vi "Main Engine Get Hardware Info.vi"(8 "error in":errorcluster) -> (0 "error out":errorcluster, 1 "CPU Session":refnum<k21>, 2 "IPAddress":string, 3 "Hardware Info":T3[](array[typedef]) {"Is Present?" items=["Initializing"=-2, "Unknown"=-1, "Not Present"=0, "Present"=1]}, 4 "DAQ Device Info":T1[](array[typedef]), 5 "Serial Device Info":T2[](array[typedef]), 6 "Ethernet IP Address":string[](array[string]), 7 "CPU Ref":refnum<k20>)   [LabVIEW 2021]
doc: "Get cRIO Info\n\n\nAll Rights Reserved © 2023 SyncSols"
uses:
  Controls/Main Engine Hardware Info Data Cluster.ctl
  Controls/Main Engine Serial Card Details.ctl
  Controls/Main Engine DAQ Device Info.ctl
  <vilib>/Instr/_visa.llb/VISA Find Search Mode.ctl
  <userlib>/_OpenG.lib/array/array.llb/Remove Duplicates from 1D Array (String)__ogtk.vi
  <vilib>/nisyscfg/nisyscfg.lvlib
  <resource>/objmgr/nicriosae.rc
  <resource>/objmgr/daqmx.rc
  <userlib>/_OpenG.lib/array/array.llb/openg_array.lvlib
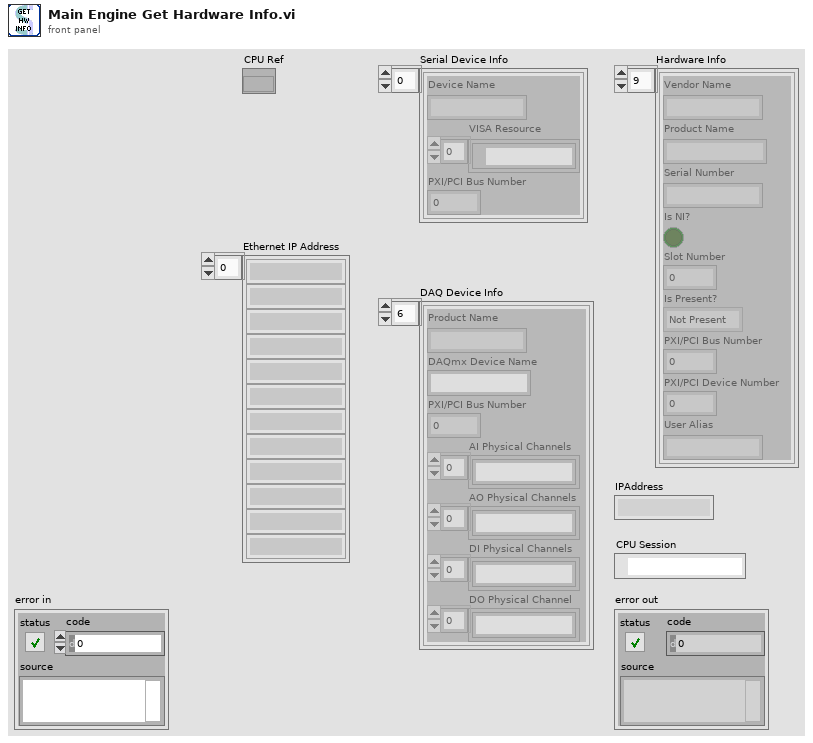
[diagram p1: front panel]
types:
  T1 = typedef "Main Engine DAQ Device Info.ctl" = cluster{"Product Name":string, "DAQmx Device Name":string, "PXI/PCI Bus Number":u32, "AI Physical Channels":string[], "AO Physical Channels":string[], "DI Physical Channels":string[], "DO Physical Channel":string[]}
  T2 = typedef "Main Engine Serial Card Details.ctl" = cluster{"Device Name":string, "VISA Resource":refnum<visa-resource-name>[], "PXI/PCI Bus Number":u32}
  T3 = typedef "Main Engine Hardware Info Data Cluster.ctl" = cluster{"Vendor Name":string, "Product Name":string, "Serial Number":string, "Is NI?":bool, "Slot Number":i32, "Is Present?":i32, "PXI/PCI Bus Number":u32, "PXI/PCI Device Number":u32, "User Alias":string}
  T4 = typedef "VISA Find Search Mode.ctl" = u32
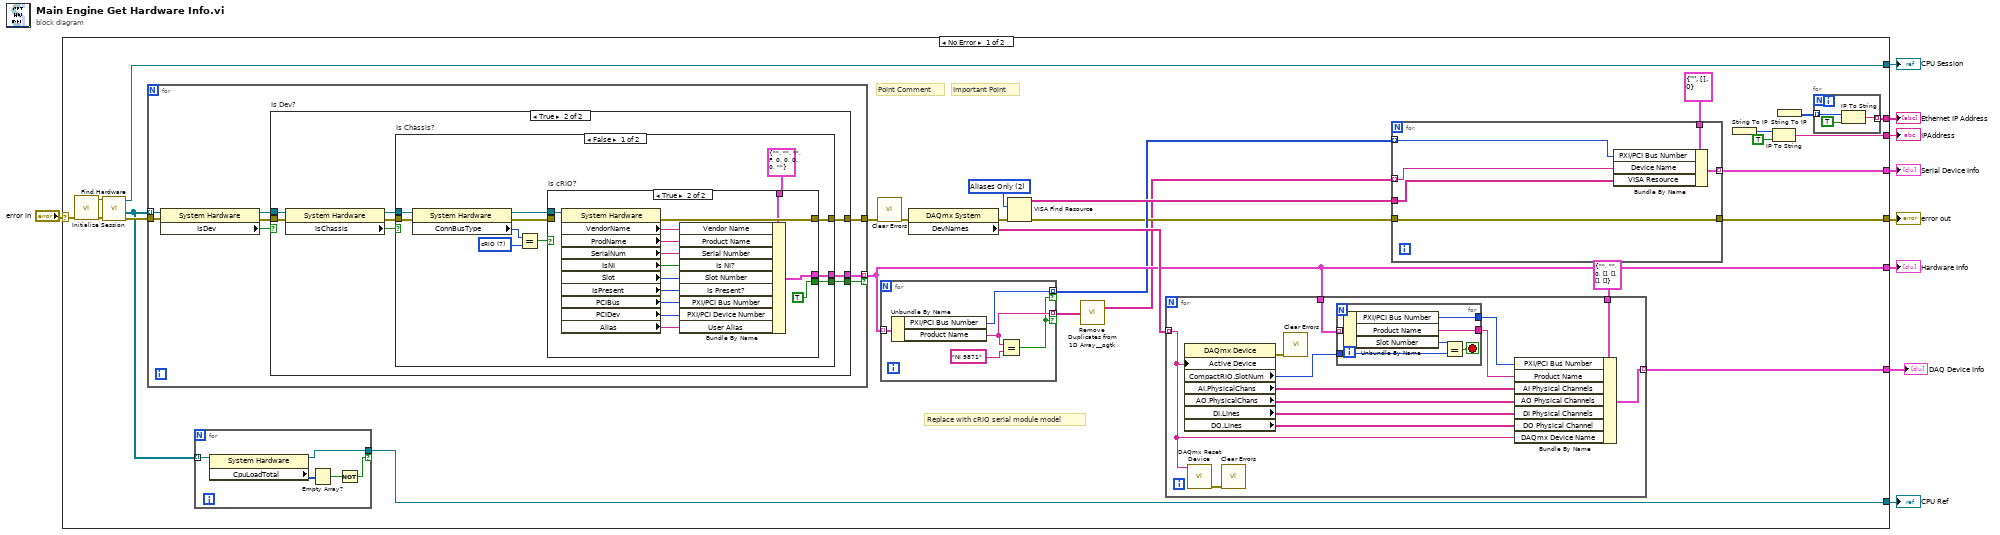
[diagram p0: block diagram]
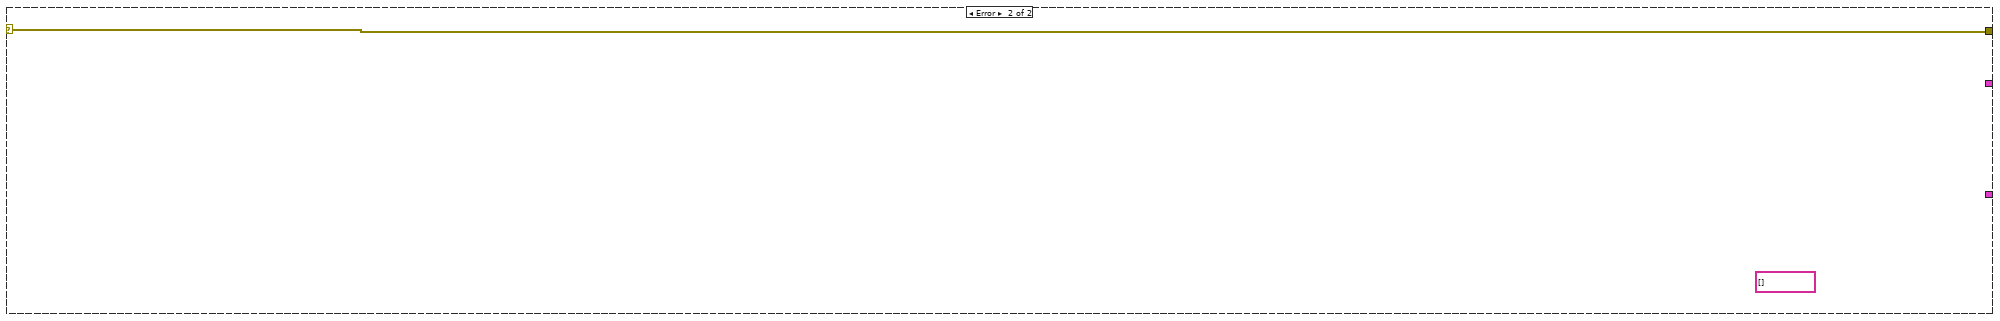
[diagram p5: hidden frame]
diagram:
  n1 = case shown="No Error" "error in" {
    selector: "error in" -> [w35 w120]
    tunnel: [w26 w120] -> w9
    tunnel: [w24 _] -> w7
    tunnel: [w33 _] -> w6
    tunnel: [w27 _] -> w5
    tunnel: [w23 _] -> w4
    tunnel: [w16 _] -> w3
    tunnel: [w15 _] -> w1
    tunnel: [w13 _] -> w2
    frame No Error {
      w29 = T4 2 items=["Canonical Names Only"=0, "Aliases Only"=2, "Include Matching Aliases"=3, "Include All Aliases"=4] ("Search Mode")
      # "Replace with cRIO serial module model"
      # "Important Point"
      # "Point Comment"
      n2 = call <vilib>:"Initialize Session.vi"("error in (no error)"=w35) -> ("error out"=w37:errorcluster, "Session out"=w36:refnum<k21>)  [unwired: 9 in]
      n3 = call <vilib>:"Find Hardware.vi"("error in (no error)"=w37, "Session in"=w36) -> ("error out"=w34:errorcluster, "Resources out"=w14:refnum<k20>[], "Session out"=w15:refnum<k21>)  [unwired: 6 in, 1 out]
      n4 = for {
        tunnel: w14 -> [w83] mode=indexing
        tunnel: w34 -> [w79]
        tunnel: [w78] -> w31
        tunnel: [w77] -> w24 mode=indexing if=w76
        n5 = property class="System Hardware"(reference=w83, error in=w79) -> (reference out=w82:refnum<k20>, error out=w81:errorcluster, "IsDev"=w80:bool)
        n6 = case "Is Dev?" shown="True" w80 {
          tunnel: w82 -> [_ w92]
          tunnel: w81 -> [w84 w91]
          tunnel: [w84 w87] -> w78
          tunnel: [_ w86] -> w76
          tunnel: [_ w85] -> w77
          frame False {
          }
          frame True {
            n7 = property class="System Hardware"(reference=w92, error in=w91) -> (reference out=w90:refnum<k20>, error out=w88:errorcluster, "IsChassis"=w89:bool)
            n8 = case "Is Chassis?" shown="False" w89 {
              tunnel: w90 -> [w103 _]
              tunnel: w88 -> [w102 w119]
              tunnel: [w97 w119] -> w87
              tunnel: [w95 _] -> w86
              tunnel: [w94 _] -> w85
              frame False {
                w100 = u32 7 items=["BuiltIn/System", "PXI/PCI", "USB", "GPIB", "VXI", "Serial", "TCP/IP", "cRIO", "SCXI", "cDAQ", "SwitchBlock", "SCC", "FireWire", "Accessory", "CAN", "SwitchBlock Device"] ("Devices & Chassis:Connects To Bus Type")
                n9 = property class="System Hardware"(reference=w103, error in=w102) -> (reference out=w96:refnum<k20>, error out=w98:errorcluster, "ConnBusType"=w101:u32)
                n10 = Equal?(x=w101, y=w100) -> (x = y?=w99:bool)
                n11 = case "Is cRIO?" shown="True" w99 {
                  tunnel: w98 -> [w104 _]
                  tunnel: [w104 w118] -> w97
                  tunnel: w96 -> [_ w107]
                  tunnel: [_ TRUE] -> w95
                  tunnel: [_ w111] -> w94
                  tunnel: T3 {"Vendor Name"="", "Product Name"="", "Serial Number"="", "Is NI?"=FALSE, "Slot Number"=0, "Is Present?"=0, "PXI/PCI Bus Number"=0, "PXI/PCI Device Number"=0, "User Alias"=""} ("Hardware Info") -> [_ w106]
                  frame False {
                  }
                  frame True {
                    n12 = property class="System Hardware"(reference=w107) -> (error out=w118:errorcluster, "VendorName"=w112:string, "ProdName"=w113:string, "SerialNum"=w114:string, "IsNI"=w115:bool, "Slot"=w108:i32, "IsPresent"=w116:i32, "PCIBus"=w110:u32, "PCIDev"=w109:u32, "Alias"=w105:string)  [unwired: 1 in, 1 out]
                    n13 = Bundle By Name(cluster=w106, "Vendor Name"=w112, "Product Name"=w113, "Serial Number"=w114, "Is NI?"=w115, "Slot Number"=w108, "Is Present?"=w116, "PXI/PCI Bus Number"=w110, "PXI/PCI Device Number"=w109, "User Alias"=w105) -> (w111:T3)
                  }
                }
              }
              frame True {
              }
            }
          }
        }
      }
      n14 = for {
        tunnel: w14 -> [w40] mode=indexing
        tunnel: [w38] -> w13 if=w39
        n15 = property class="System Hardware"(reference=w40) -> (reference out=w38:refnum<k20>, "CpuLoadTotal"=w42:u32[])  [unwired: 1 in, 1 out]
        n16 = Empty Array?(array=w42) -> (empty?=w41:bool)
        n17 = Not(x=w41) -> (.not. x?=w39:bool)
      }
      n18 = call <vilib>:"Clear Errors.vi"("error in (no error)"=w31) -> ("error out"=w12:errorcluster)  [unwired: 5 in, 1 out]
      n19 = for {
        tunnel: w24 -> [w69] mode=indexing
        tunnel: [w67] -> w11 mode=indexing if=w65
        tunnel: [w68] -> w22 mode=indexing if=w65
        n20 = Unbundle By Name(w69) -> ("PXI/PCI Bus Number"=w68:u32, "Product Name"=w67:string)
        n21 = Equal?(x=w67, y="NI 9871") -> (x = y?=w65:bool)
      }
      n22 = property class="DAQmx System"(error in=w12) -> (error out=w30:errorcluster, "DevNames"=w25:tag[])  [unwired: 1 in, 1 out]
      n23 = VISA Find Resource(8:w30, 10:w29) -> (0:w19:errorcluster, 3:w28:string[])  [unwired: 1 in, 1 out]
      n24 = call-poly <userlib>:"Remove Duplicates from 1D Array__ogtk.vi"("Input Array"=w11) -> ("Output Array"=w10:string[])  [unwired: 1 out]
      n25 = for {
        tunnel: w25 -> [w46] mode=indexing
        tunnel: w24 -> [w58]
        tunnel: [w55] -> w23 mode=indexing
        tunnel: T1 {"Product Name"="", "DAQmx Device Name"="", "PXI/PCI Bus Number"=0, "AI Physical Channels"=[], "AO Physical Channels"=[], "DI Physical Channels"=[], "DO Physical Channel"=[]} ("Daq Device Info") -> [w53]
        n26 = property class="DAQmx Device"("Active Device"=w46) -> (error out=w48:errorcluster, "CompactRIO.SlotNum"=w57:u32, "AI.PhysicalChans"=w52:tag[], "AO.PhysicalChans"=w51:tag[], "DI.Lines"=w50:tag[], "DO.Lines"=w49:tag[])  [unwired: 2 in, 1 out]
        n27 = call <vilib>:"DAQmx Reset Device.vi"("device in"=w46) -> ("error out"=w47:errorcluster)  [unwired: 14 in]
        n28 = call <vilib>:"Clear Errors.vi"("error in (no error)"=w47) -> ()  [unwired: 5 in, 2 out]
        n29 = call <vilib>:"Clear Errors.vi"("error in (no error)"=w48) -> ()  [unwired: 5 in, 2 out]
        n30 = for {
          tunnel: w58 -> [w64] mode=indexing
          tunnel: w57 -> [w59]
          tunnel: [w63] -> w56
          tunnel: [w61] -> w54
          stop <- w62 stop-if-true
          n31 = Unbundle By Name(w64) -> ("PXI/PCI Bus Number"=w63:u32, "Product Name"=w61:string, "Slot Number"=w60:i32)
          n32 = Equal?(x=w60, y=w59) -> (x = y?=w62:bool)
        }
        n33 = Bundle By Name(cluster=w53, "PXI/PCI Bus Number"=w56, "Product Name"=w54, "AI Physical Channels"=w52, "AO Physical Channels"=w51, "DI Physical Channels"=w50, "DO Physical Channel"=w49, "DAQmx Device Name"=w46) -> (w55:T1)
      }
      n34 = for {
        tunnel: w10 -> [w75] mode=indexing
        tunnel: w28 -> [w74]
        tunnel: w19 -> [w70]
        tunnel: [w73] -> w27 mode=indexing
        tunnel: [w70] -> w26
        tunnel: w22 -> [w71] mode=indexing
        tunnel: T2 {"Device Name"="", "VISA Resource"=[], "PXI/PCI Bus Number"=0} ("Serial Details") -> [w72]
        n35 = Bundle By Name(cluster=w72, "PXI/PCI Bus Number"=w71, "Device Name"=w75, "VISA Resource"=w74) -> (w73:T2)
      }
      n36 = String To IP() -> (0:w18:u32)  [unwired: 1 in]
      n37 = IP To String(1:TRUE ("dot notation? (F)"), 2:w18) -> (0:w33:string)
      n38 = String To IP() -> (0:w17:u32[])  [unwired: 1 in]
      n39 = for {
        tunnel: w17 -> [w43] mode=indexing
        tunnel: [w44] -> w16 mode=indexing
        n40 = IP To String(1:TRUE ("dot notation? (F)"), 2:w43) -> (0:w44:string)
      }
    }
    frame Error {
      (unwired) tag[] []
    }
  }
  "error out" <- w9
  "Hardware Info" <- w7
  "IPAddress" <- w6
  "Serial Device Info" <- w5
  "DAQ Device Info" <- w4
  "Ethernet IP Address" <- w3
  "CPU Ref" <- w2
  "CPU Session" <- w1
